vi "FGV_ThreadsManager.vi"(7 "Action":T1, 8 "error in":errorcluster caption="错误输入（无错误）", 10 "Tag":string) -> (0 "error out":errorcluster caption="错误输出", 2 "Vi*":refnum<vi>)   [LabVIEW 2016]
uses:
  FGV_ThreadsManager.ctl
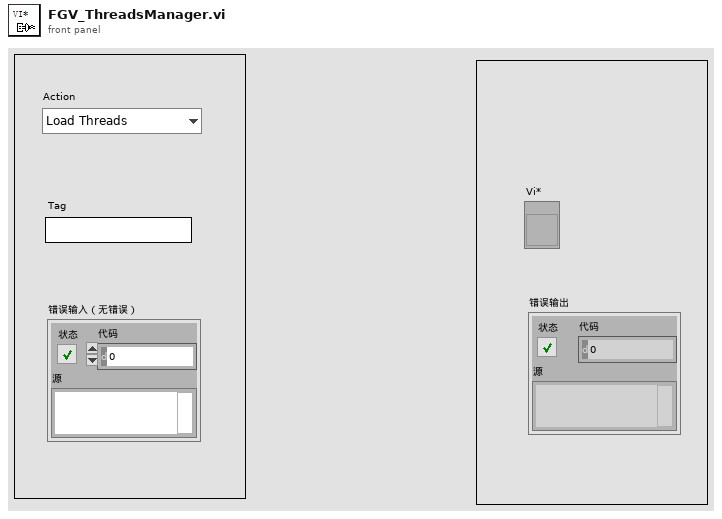
[diagram p1: front panel]
types:
  T1 = typedef "FGV_ThreadsManager.ctl" = enum16{"Load Threads", "GetVI*", "Other"}
  T2 = cluster{"TREE PNG":path, "User Guide":path, "DefaultSave":path, "BuildPath":path, "Image":path, "Modules":path, "Configuration":path, "License":path, "SplitFiles":path, "System.ini":path}
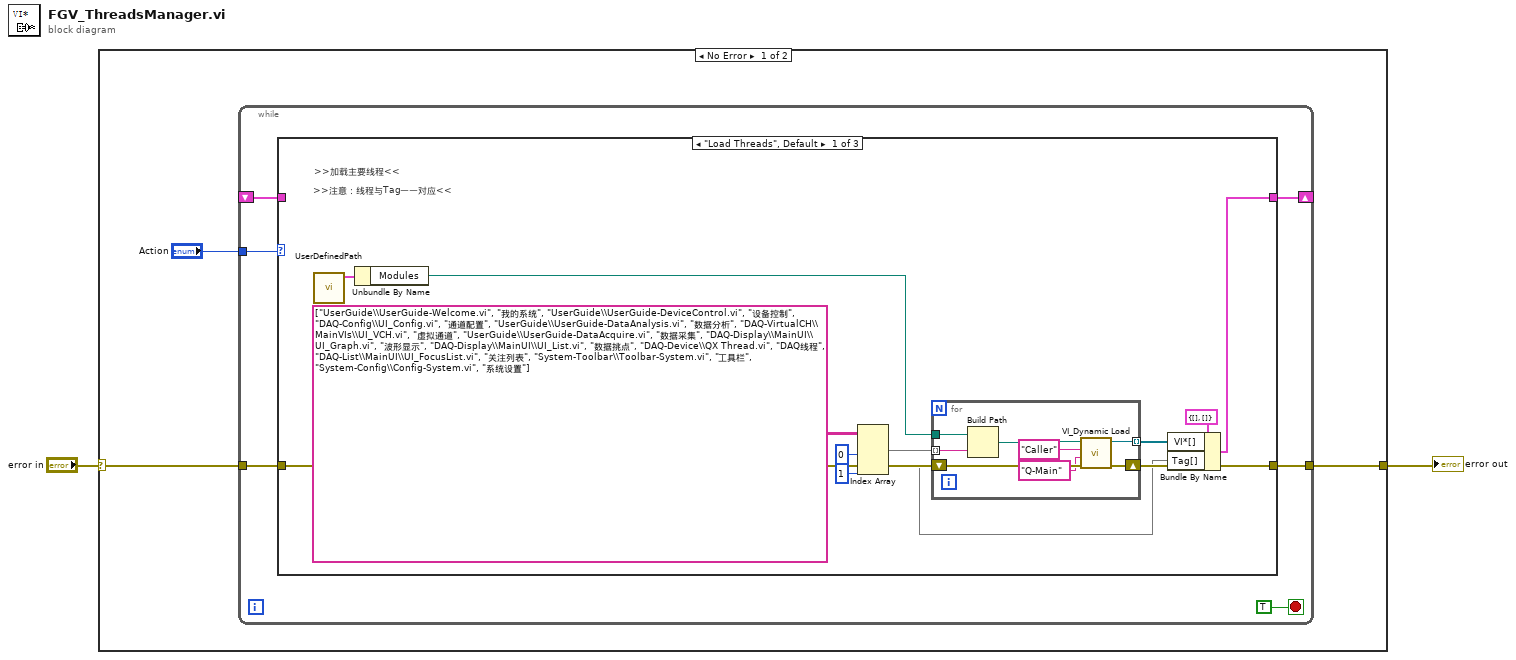
[diagram p0: block diagram]
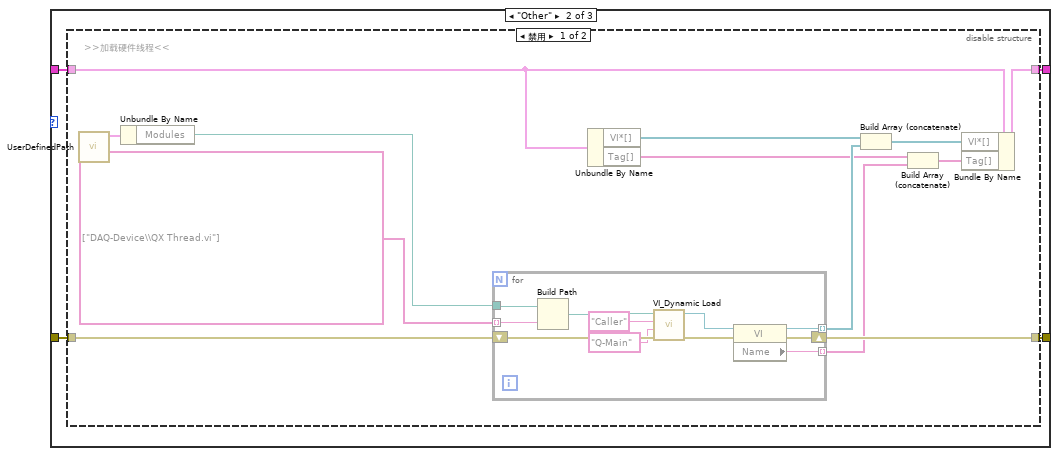
[diagram p2: hidden frame]
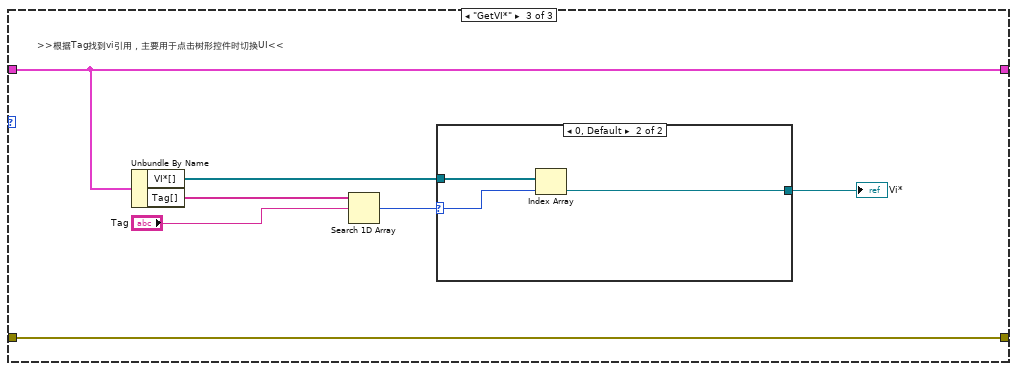
[diagram p4: hidden frame]
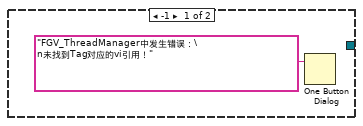
[diagram p5: hidden frame]
diagram:
  n1 = case shown="No Error" "error in" {
    selector: "error in" -> [w4 w73]
    tunnel: [w3 w73] -> w1
    frame No Error {
      n2 = while {
        shift-right: [w9] -> _
        shift-left: _ -> [w8]
        tunnel: "Action" -> [w10]
        tunnel: w4 -> [w7]
        tunnel: [w6] -> w3
        stop <- TRUE stop-if-true
        n3 = case shown="\"Load Threads\", Default" w10 {
          tunnel: [w22 w35 w67] -> w9
          tunnel: w8 -> [_ w32 w67]
          tunnel: w7 -> [w20 w34 w68]
          tunnel: [w17 w33 w68] -> w6
          frame "Load Threads", Default {
            # ">>注意：线程与Tag一一对应<<"
            # ">>加载主要线程<<"
            n4 = call "UserDefinedPath.vi"() -> ("UserDefinedPath"=w19:T2)  [unwired: 11 in]
            n5 = Unbundle By Name(w19) -> ("Modules"=w18:path)
            n6 = Index Array(array=string[][] [["UserGuide\\UserGuide-Welcome.vi", "我的系统"], ["UserGuide\\UserGuide-DeviceControl.vi", "设备控制"], ["DAQ-Config\\UI_Config.vi", "通道配置"], ["UserGuide\\UserGuide-DataAnalysis.vi", "数据分析"], ["DAQ-VirtualCH\\MainVIs\\UI_VCH.vi", "虚拟通道"], ["UserGuide\\UserGuide-DataAcquire.vi", "数据采集"], ["DAQ-Display\\MainUI\\UI_Graph.vi", "波形显示"], ["DAQ-Display\\MainUI\\UI_List.vi", "数据挑点"], ["DAQ-Device\\QX Thread.vi", "DAQ线程"], ["DAQ-List\\MainUI\\UI_FocusList.vi", "关注列表"], ["System-Toolbar\\Toolbar-System.vi", "工具栏"], ["System-Config\\Config-System.vi", "系统设置"]] ("转置的数组"), index (col) #1=0 ("禁用的索引 (列)"), index (col) #2=1 ("索引 (列)")) -> (element #1=w16:string[], element #2=w12:string[])  [unwired: 2 in]
            n7 = for {
              shift-right: [w30] -> w17
              shift-left: w20 -> [w31]
              tunnel: [w29] -> w21 mode=indexing
              tunnel: w18 -> [w26]
              tunnel: w16 -> [w24] mode=indexing
              n8 = Build Path(base path=w26, name or relative path=w24) -> (appended path=w25:path)
              n9 = call "VI_Dynamic Load.vi"("error in"=w31, "CtrlValue"="Q-Main" ("CtrlName"), "CtrlName"="Caller", "Vi Path"=w25) -> ("错误输出"=w30:errorcluster, "vi reference"=w29:refnum<vi>)  [unwired: 6 in]
            }
            n10 = Bundle By Name(cluster=cluster{"VI*[]":refnum<vi>[], "Tag[]":string[]} {"VI*[]"=[], "Tag[]"=[]} ("Data"), "VI*[]"=w21, "Tag[]"=w12) -> (w22:cluster{"VI*[]":refnum<vi>[], "Tag[]":string[]})
          }
          frame "Other" {
            n11 = disable-structure shown="禁用" {
              disable-tunnel: [w48 w61] -> w35
              disable-tunnel: w34 -> [w47 w60]
              disable-tunnel: [w46 w60] -> w33
              disable-tunnel: w32 -> [w42 w61]
              frame Disabled {
                # ">>加载硬件线程<<"
                n12 = call "UserDefinedPath.vi"() -> ("UserDefinedPath"=w45:T2)  [unwired: 11 in]
                n13 = Unbundle By Name(w45) -> ("Modules"=w43:path)
                n14 = for {
                  shift-right: [w51] -> w46
                  shift-left: w47 -> [w59]
                  tunnel: [w49] -> w40 mode=indexing
                  tunnel: string[] ["DAQ-Device\\QX Thread.vi"] -> [w55] mode=indexing
                  tunnel: w43 -> [w54]
                  tunnel: [w50] -> w37 mode=indexing
                  n15 = Build Path(base path=w54, name or relative path=w55) -> (appended path=w56:path)
                  n16 = call "VI_Dynamic Load.vi"("error in"=w59, "CtrlValue"="Q-Main" ("CtrlName"), "CtrlName"="Caller", "Vi Path"=w56) -> ("错误输出"=w52:errorcluster, "vi reference"=w53:refnum<vi>)  [unwired: 6 in]
                  n17 = property class="VI"(reference=w53, error in=w52) -> (reference out=w49:refnum<vi>, error out=w51:errorcluster, "Name"=w50:string)
                }
                n18 = Unbundle By Name(w42) -> ("VI*[]"=w41:refnum<vi>[], "Tag[]"=w38:string[])
                n19 = Build Array (concatenate)(w41, w40) -> (w39:refnum<vi>[])
                n20 = Build Array (concatenate)(w38, w37) -> (w36:string[])
                n21 = Bundle By Name(cluster=w42, "VI*[]"=w39, "Tag[]"=w36) -> (w48:cluster{"VI*[]":refnum<vi>[], "Tag[]":string[]})
              }
              frame Enabled {
              }
            }
          }
          frame "GetVI*" {
            # ">>根据Tag找到vi引用，主要用于点击树形控件时切换UI<<"
            n22 = Unbundle By Name ("按名称解除捆绑")(w67) -> ("VI*[]"=w64:refnum<vi>[], "Tag[]"=w66:string[])
            n23 = Search 1D Array ("搜索一维数组")(1D array=w66, element="Tag") -> (index of element=w63:i32)  [unwired: 1 in]
            n24 = case "条件结构" shown="0, Default" w63 {
              selector: w63 -> [_ w71]
              tunnel: w64 -> [_ w72]
              tunnel: [_ w70] -> w62
              frame -1 {
                n25 = One Button Dialog(message="FGV_ThreadManager中发生错误：\n未找到Tag对应的vi引用！" ("消息")) -> ()  [unwired: 1 in, 1 out]
              }
              frame 0, Default {
                n26 = Index Array(array=w72, index=w71) -> (element=w70:refnum<vi>)
              }
            }
            "Vi*" <- w62
          }
        }
      }
    }
    frame Error {
    }
  }
  "error out" <- w1
